vi "Error announcer - CTI.vi"(3 "error in (no error)":errorcluster, 5 "2 button dialog? (F)":bool) -> (2 "Exit?":bool)   [LabVIEW 2013]
doc: "If error in = T, this vi announces the error and error code."
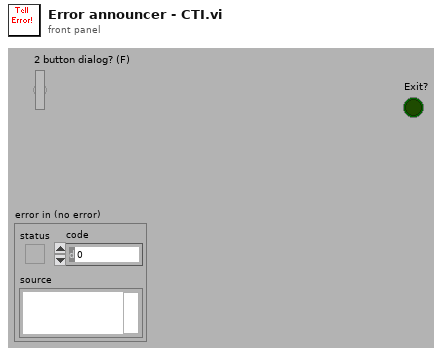
[diagram p1: front panel]
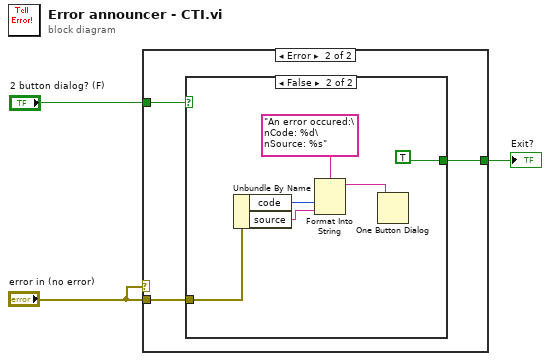
[diagram p0: block diagram]
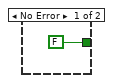
[diagram p2: hidden frame]
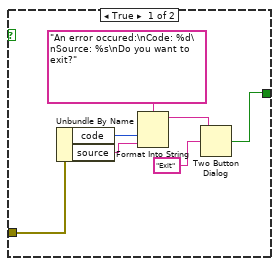
[diagram p3: hidden frame]
diagram:
  n1 = case shown="Error" "error in (no error)" {
    tunnel: "error in (no error)" -> [_ w7]
    tunnel: "2 button dialog? (F)" -> [_ w6]
    tunnel: [FALSE w5] -> w1
    frame No Error {
    }
    frame Error {
      n2 = case shown="False" w6 {
        tunnel: w7 -> [w10 w16]
        tunnel: [w9 TRUE] -> w5
        frame True {
          n3 = Unbundle By Name(w10) -> ("code"=w14:i32, "source"=w13:string)
          n4 = Format Into String(format string="An error occured:\nCode: %d\nSource: %s\nDo you want to exit?", w14, w13) -> (resulting string=w12:string)  [unwired: 2 in, 1 out]
          n5 = Two Button Dialog(message=w12, 2:"Exit" ("T button name (\"OK\")")) -> (T button?=w9:bool)  [unwired: 1 out]
        }
        frame False {
          n6 = Unbundle By Name(w16) -> ("code"=w20:i32, "source"=w19:string)
          n7 = Format Into String(format string="An error occured:\nCode: %d\nSource: %s", w20, w19) -> (resulting string=w18:string)  [unwired: 2 in, 1 out]
          n8 = One Button Dialog(message=w18) -> ()  [unwired: 2 out]
        }
      }
    }
  }
  "Exit?" <- w1
